vi "빌드대상.vi"() -> ()   [LabVIEW 2014]
panel:
  out "웨이브폼 차트":dbl(graph)
  in  "정지":bool
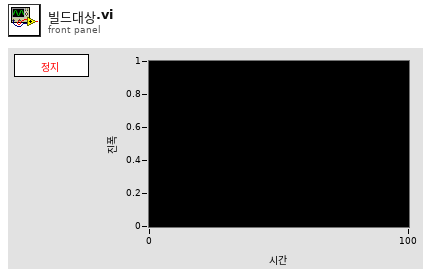
[diagram p1: front panel]
types:
  T1 = enum32{"invalid app kind", "Development System", "Run Time System", "Student Edition", "Embedded LabVIEW", "Evaluation", "Custom"}
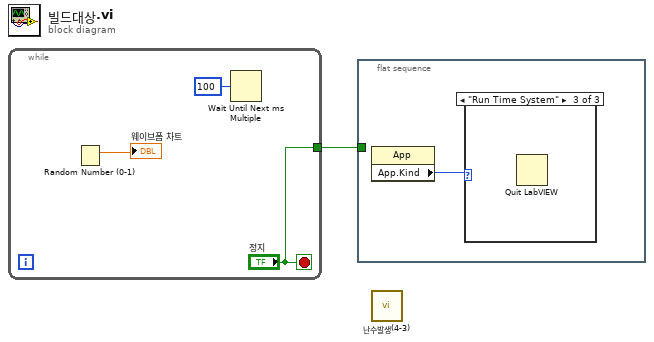
[diagram p0: block diagram]
diagram:
  n1 = while {
    tunnel: ["정지"] -> w1
    stop <- "정지" stop-if-true
    n2 = Random Number (0-1)() -> (number: 0 to 1=→"웨이브폼 차트":dbl)
    n3 = Wait Until Next ms Multiple(millisecond multiple=u32 100 ("ms 배수")) -> ()  [unwired: 1 out]
  }
  n4 = flat-sequence {
    tunnel: w1 -> [_]
    frame #0 {
      n5 = property class="App"() -> ("App.Kind"=w5:T1)  [unwired: 2 in, 2 out]
      n6 = case shown="\"Run Time System\"" w5 {
        frame "invalid app kind", Default {
        }
        frame "Development System" {
        }
        frame "Run Time System" {
          n7 = Quit LabVIEW() -> ()  [unwired: 1 in]
        }
      }
    }
  }
  n8 = call "난수발생(4-3).vi"() -> ()  [unwired: 12 in]
